vi "FpgaLink_Read_Channel.vi"(6 "Timeout (10000)":u32=10000, 8 "error in (no error)":errorcluster, 9 "Count":u32, 10 "Channel":u8, 11 "handle":i64) -> (0 "error out":errorcluster, 2 "data":u8[](array[numeric]), 3 "handle out":i64)   [LabVIEW 2011]
doc: "Read the specified channel into the supplied buffer.\n\nRead count bytes from the FPGA channel chan to the data array, with the given timeout in milliseconds. In the event of a timeout, the connection between host and FPGA will be left in an undefined state; before the two can resynchronise it's likely the FPGA will need to be reset and the host side disconnected (flOpen()) and reconnected (flClose()) again. Before calling flReadChannel(), you should verify that the FPGALink device actually supports CommFPGA using flIsCommCapable()."
uses:
  <vilib>/Utility/importsl/GetValueByPointer/datatype.ctl
  <vilib>/Utility/importsl/GetValueByPointer/GetValueByPointer.xnode
  resource/lvimptsl.dll
  libfpgalink.dll
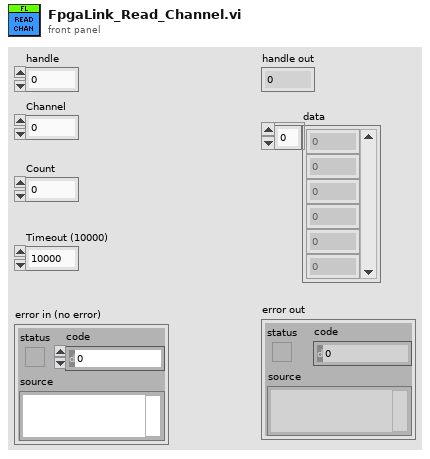
[diagram p1: front panel]
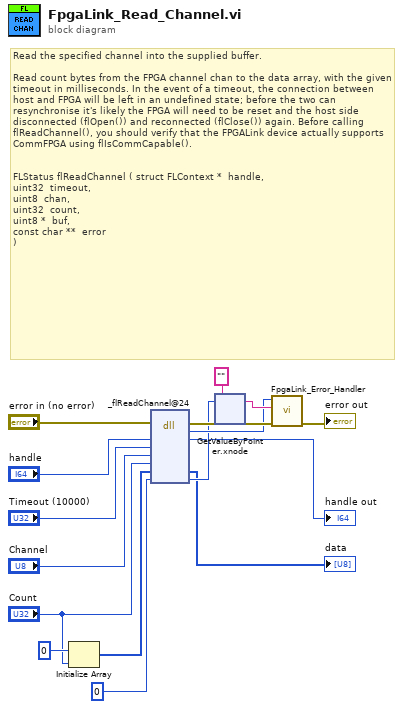
[diagram p0: block diagram]
diagram:
  # "Read the specified channel into the supplied buffer.\n\nRead count bytes from the FPGA channel chan to the data array, with the given timeout in milliseconds. In the event of a timeout, the connection between host and FPGA will be left in an undefined state; before the two can resynchronise it's likely the FPGA will need to be reset and the host side disconnected (flOpen()) and reconnected (flClose()) again. Before calling flReadChannel(), you should verify that the FPGALink device actually supports CommFPGA using flIsCommCapable().\n\n\nFLStatus flReadChannel\t(\tstruct FLContext * \thandle,\nuint32 \ttimeout,\nuint8 \tchan,\nuint32 \tcount,\nuint8 * \tbuf,\nconst char ** \terror \n)"
  n1 = Initialize Array(u8 0 ("chan"), "Count") -> (w3:u8[])
  n2 = dll-call lib="libfpgalink.*" fn="_flReadChannel@24"(error in="error in (no error)", "handle"="handle", "timeout"="Timeout (10000)", "chan"="Channel", "count"="Count", "buf"=w3, "error"=i64 0) -> (error out=w10:errorcluster, "FLStatus"=w9:u32, "handle"=→"handle out":i64, "buf"=→"data":u8[], "error"=w8:i64)  [unwired: 5 in, 1 out]
  n3 = xnode "GetValueByPointer.xnode"("Pointer"=w8, "InputType"="", "ErrorIn"=w10) -> ("Output"=w12:string, "ErrorOut"=w14:errorcluster)  [unwired: 1 in]
  n4 = call <vilib>:"FpgaLink_Error_Handler.vi"("error in (no error)"=w14, "error string"=w12, "error code"=w9) -> ("error out"=→"error out":errorcluster)  [unwired: 8 in]
